vi "ConnectSimple.vi"(4 "Show Protocol":bool=TRUE, 6 "Interface (1: RS232; 2: ArcNet; 3: DPRAM)":u32=1, 7 "Baudrate":u16=9600, 8 "error in (no error)":errorcluster, 9 "I/O Adress (DPRAM)":u32=832 format="%.0x", 10 "COM Port":u32=1, 11 "DelayLineLS4 in":refnum<class "DLLS4.lvclass">) -> (0 "error out":errorcluster, 3 "DelayLineLS4 out":refnum<class "DLLS4.lvclass">)   [LabVIEW 2015, in "DLLS4.lvclass"]
uses:
  DLLS4.lvclass
  DelayLine.lvclass/DelayLine.ctl
  <vilib>/Utility/error.llb/DialogType.ctl
  <vilib>/ErrorRing/Error Ring.xnode
  DelayLine.lvclass
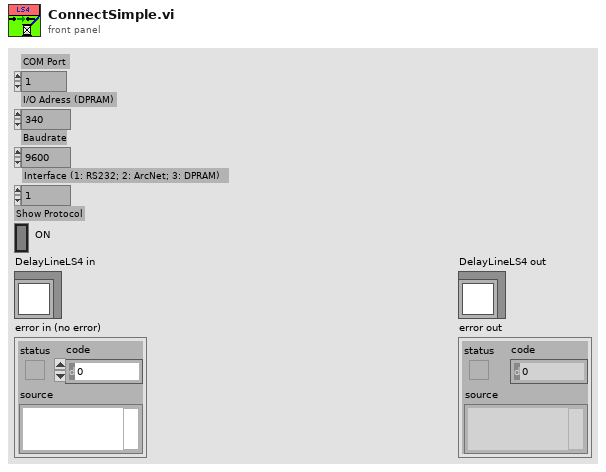
[diagram p1: front panel]
types:
  T1 = typedef "DialogType.ctl" = u16
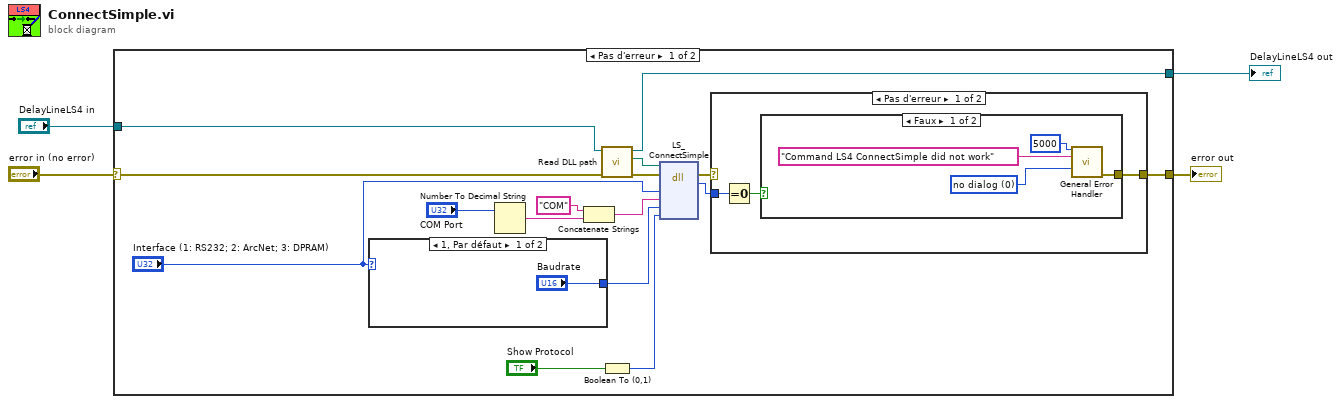
[diagram p0: block diagram]
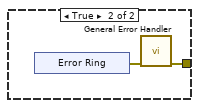
[diagram p2: hidden frame]
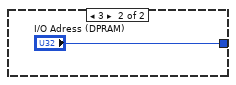
[diagram p4: hidden frame]
diagram:
  n1 = case shown="Pas d'erreur" "error in (no error)" {
    selector: "error in (no error)" -> [w8 w35]
    tunnel: [w10 w35] -> w3
    tunnel: [w5 w34] -> w1
    tunnel: "DelayLineLS4 in" -> [w9 w34]
    frame No Error {
      n2 = case shown="1, Par défaut" "Interface (1: RS232; 2: ArcNet; 3: DPRAM)" {
        tunnel: ["Baudrate" "I/O Adress (DPRAM)"] -> w15
        frame 1, Default {
        }
        frame 3 {
        }
      }
      n3 = Number To Decimal String(number="COM Port") -> (decimal integer string=w13:string)  [unwired: 1 in]
      n4 = Concatenate Strings("COM", w13) -> (w11:string)
      n5 = call "Read DLL path.vi"("error in (no error)"=w8, "DelayLine in"=w9) -> ("error out"=w7:errorcluster, "DLL path"=w6:path, "DelayLine out"=w5:refnum<class "DLLS4.lvclass">)  [unwired: 7 in]
      n6 = Boolean To (0,1)(Boolean="Show Protocol") -> (0, 1=w18:i16)
      n7 = dll-call lib="S:/TRANCON/DLL/LStep4.dll" fn="LS_ConnectSimple" ("Call Library Function")(path in=w6, error in=w7, "AnInterfaceType"="Interface (1: RS232; 2: ArcNet; 3: DPRAM)", "AComName"=w11, "ABR"=w15, "AShowProt"=w18) -> (error out=w20:errorcluster, "type de retour"=w19:i32)  [unwired: 5 in, 1 out]
      n8 = case shown="Pas d'erreur" w20 {
        selector: w20 -> [_ w31]
        tunnel: w19 -> [w23 _]
        tunnel: [w21 w31] -> w10
        frame No Error {
          n9 = Equal To 0?(x=w23) -> (x = 0?=w22:bool)
          n10 = case shown="Faux" w22 {
            tunnel: [w25 w28] -> w21
            frame False {
              w24 = T1 0 items=["no dialog", "OK message", "continue or stop message", "OK message + warnings", "continue/stop + warnings"] ("type of dialog (OK msg:1)")
              n11 = call <vilib>:"General Error Handler.vi"("[error code] (0)"=5000 ("code"), "[error source] (\" \")"="Command LS4 ConnectSimple did not work" ("String to Prepend to source (\"\")"), "type of dialog (OK msg:1)"=w24) -> ("error out"=w25:errorcluster)  [unwired: 8 in, 4 out]
            }
            frame True {
              n12 = xnode "Error Ring"() -> ("sortie d'erreur"=w29:errorcluster)
              n13 = call <vilib>:"General Error Handler.vi"("error in (no error)"=w29) -> ("error out"=w28:errorcluster)  [unwired: 10 in, 4 out]
            }
          }
        }
        frame Error {
        }
      }
    }
    frame Error {
    }
  }
  "error out" <- w3
  "DelayLineLS4 out" <- w1
